vi "Gear Ratio (Drive).vi"(10 "Wheel size (in)":dbl, 11 "Gear ratio":dbl) -> (2 "Position Factor":dbl, 3 "Velocity Factor (ft/s)":dbl)   [LabVIEW 2025]
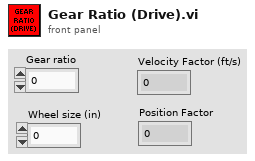
[diagram p1: front panel]
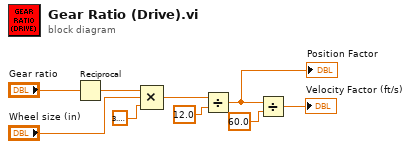
[diagram p0: block diagram]
diagram:
  n1 = Reciprocal(x="Gear ratio") -> (1/x=w8:dbl)
  n2 = Compound Arithmetic op=MULTIPLY(w8, "Wheel size (in)", 3.141592653589793) -> (w5:dbl)
  n3 = Divide(x=w5, y=12.0) -> (x/y=w2:dbl)
  "Position Factor" <- w2
  n4 = Divide(x=w2, y=60.0) -> (x/y=→"Velocity Factor (ft/s)":dbl)
